vi "Day 22-Pasre Data.vi"(11 "Data in":string[][](array[string])) -> (3 "Instructions out":cluster{i64[], i64}[](array[cluster]))   [LabVIEW 2021]
uses:
  <vilib>/regexp/Match Regular Expression.xnode
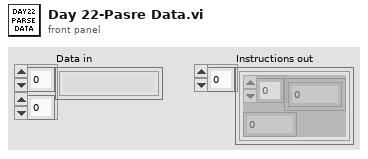
[diagram p1: front panel]
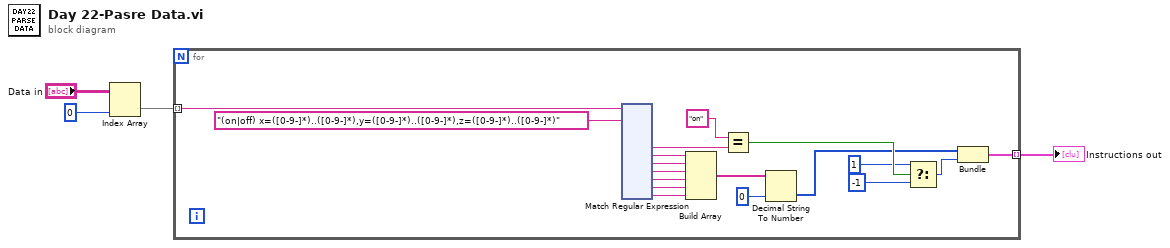
[diagram p0: block diagram]
diagram:
  n1 = Index Array(array="Data in", index (col)=0 ("disabled index (col)")) -> (element=w1:string[])  [unwired: 1 in]
  n2 = for {
    tunnel: w1 -> [w22] mode=indexing
    tunnel: [w5] -> w4 mode=indexing
    n3 = xnode "Match Regular Expression"("input string"=w22, "regular expression"="(on|off) x=([0-9-]*)..([0-9-]*),y=([0-9-]*)..([0-9-]*),z=([0-9-]*)..([0-9-]*)") -> ("submatch 1"=w20:string, "submatch 2"=w18:string, "submatch 3"=w17:string, "submatch 4"=w16:string, "submatch 5"=w15:string, "submatch 6"=w14:string, "submatch 7"=w13:string)  [unwired: 4 in, 5 out]
    n4 = Build Array(w18, w17, w16, w15, w14, w13) -> (w12:string[])
    n5 = Equal?(x="on", y=w20) -> (x = y?=w10:bool)
    n6 = Decimal String To Number(string=w12, default (0L)=i64 0 ("default (0 I32)")) -> (number=w7:i64[])  [unwired: 1 in, 1 out]
    n7 = Select(t=i64 1, s=w10, f=i64 -1) -> (s? t:f=w6:i64)
    n8 = Bundle(w7, w6) -> (w5:cluster{i64[], i64})  [unwired: 1 in]
  }
  "Instructions out" <- w4
